vi "WFDC Messenger Template.vi"() -> (15 "Error Out":errorcluster)   [LabVIEW 2020]
uses:
  <vilib>/vision/Image Controls.llb/IMAQ Image.ctl
  WFDC Controls/WFDC Actions.ctl
  WFDC Controls/WFDC Notifier Element.ctl
  WFDC Controls/WFDC Status.ctl
  WFDC Controls/WFDC Cycle Pause.ctl
  WFDC Controls/WFDC External Sync.ctl
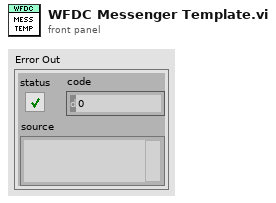
[diagram p1: front panel]
types:
  T1 = typedef "WFDC Notifier Element.ctl" = cluster{"WFDC Actions":T2, "Initial XYZ Positions":dbl[], "Ref Images":T3[], "Calibration (slope, inter)":dbl[], "Base Path":path, "Latest Scan Path":path, "Error":errorcluster, "XYZ Drift":dbl[]}
  T2 = typedef "WFDC Actions.ctl" = enum16{"Error Check", "Remote Start", "Move to Pos", "Pre Start Get Drift", "Pre Start Check Drift", "Pre Start Z Drift", "Pre Start XY Drift", "Pre Start ReFocus", "Setup New DC", "Setup Camera", "Get Ref Images", "Calc Calibration", "Switch Tabs", "Get Drift", "Z Drift", "XY Drift", "Start Cycle", "Stop DC", "Abort Remote", "Exit Loop", "Set Error", "Generate Calibration", "Quit"}
  T3 = typedef "IMAQ Image.ctl" = refnum<image>
  T4 = typedef "WFDC External Sync.ctl" = cluster{"Cycle Sync":T5, "Z Offset":dbl, "WFDC Status":T6}
  T5 = typedef "WFDC Cycle Pause.ctl" = enum16{"Pause Requested", "Paused", "Resume Requested", "Resumed"}
  T6 = typedef "WFDC Status.ctl" = enum16{"Idle", "Busy", "DC Active", "Error", "Canceled"}
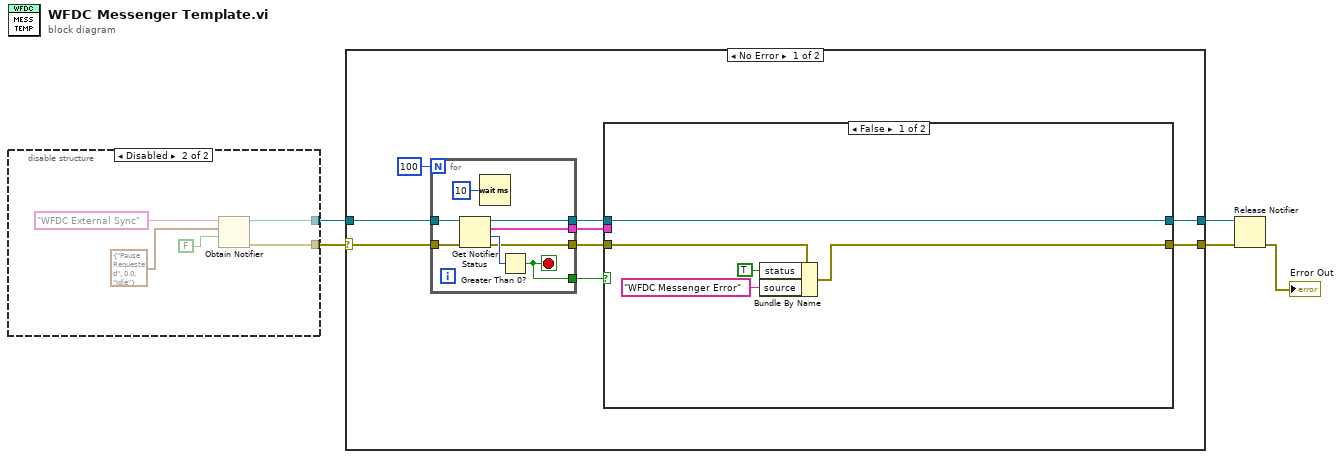
[diagram p0: block diagram]
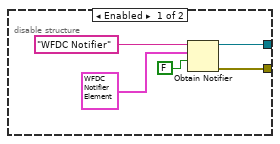
[diagram p2: hidden frame]
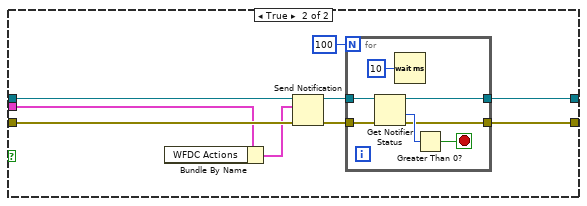
[diagram p3: hidden frame]
diagram:
  n1 = disable-structure shown="Disabled" {
    disable-tunnel: [w7 w12] -> w2
    disable-tunnel: [w6 w11] -> w1
    frame Enabled {
      n2 = Obtain Notifier(name (unnamed)="WFDC Notifier", notification data type=T1 {"WFDC Actions"=enum."Error Check", "Initial XYZ Positions"=[], "Ref Images"=[], "Calibration (slope, inter)"=[], "Base Path"=path "", "Latest Scan Path"=path "", "Error"={"status"=FALSE, "code"=0, "source"=""}, "XYZ Drift"=[]} ("WFDC Notifier Element"), create if not found? (T)=FALSE) -> (notifier out=w7:refnum<notifier>, error out=w6:errorcluster)  [unwired: 1 in, 1 out]
    }
    frame Disabled {
      n3 = Obtain Notifier(name (unnamed)="WFDC External Sync", notification data type=T4 {"Cycle Sync"=enum."Pause Requested", "Z Offset"=0.0, "WFDC Status"=enum."Idle"} ("WFDC External Sync"), create if not found? (T)=FALSE) -> (notifier out=w12:refnum<notifier>, error out=w11:errorcluster)  [unwired: 1 in, 1 out]
    }
  }
  n4 = case shown="No Error" w1 {
    selector: w1 -> [w22 w54]
    tunnel: w2 -> [w23 w55]
    tunnel: [w17 w55] -> w5
    tunnel: [w16 w54] -> w4
    frame No Error {
      n5 = for {
        N: 100 -> [_]
        tunnel: w23 -> [w52]
        tunnel: w22 -> [w51]
        tunnel: [w49] -> w20
        tunnel: [w48] -> w19
        tunnel: [w47] -> w21
        tunnel: [w46] -> w18
        stop <- w47 stop-if-true
        n6 = Get Notifier Status(notifier=w52, error in (no error)=w51) -> (notifier out=w49:refnum<notifier>, current notification=w46:T1, # waiting=w50:i32, error out=w48:errorcluster)  [unwired: 1 out]
        n7 = Wait (ms)(milliseconds to wait=u32 10) -> ()  [unwired: 1 out]
        n8 = Greater Than 0?(x=w50) -> (x > 0?=w47:bool)
      }
      n9 = case shown="False" w21 {
        tunnel: w20 -> [w29 w38]
        tunnel: w19 -> [w28 w37]
        tunnel: w18 -> [_ w31]
        tunnel: [w29 w33] -> w17
        tunnel: [w25 w32] -> w16
        frame False {
          n10 = Bundle By Name(cluster=w28, "status"=TRUE, "source"="WFDC Messenger Error") -> (w25:errorcluster)
        }
        frame True {
          n11 = Bundle By Name(cluster=w31) -> (w30:T1)  [unwired: 1 in]
          n12 = Send Notification(notification=w30, notifier=w38, error in (no error)=w37) -> (notifier out=w35:refnum<notifier>, error out=w34:errorcluster)
          n13 = for {
            N: 100 -> [_]
            tunnel: w35 -> [w44]
            tunnel: w34 -> [w43]
            tunnel: [w41] -> w33
            tunnel: [w40] -> w32
            stop <- w39 stop-if-true
            n14 = Get Notifier Status(notifier=w44, error in (no error)=w43) -> (notifier out=w41:refnum<notifier>, # waiting=w42:i32, error out=w40:errorcluster)  [unwired: 2 out]
            n15 = Wait (ms)(milliseconds to wait=u32 10) -> ()  [unwired: 1 out]
            n16 = Greater Than 0?(x=w42) -> (x > 0?=w39:bool)
          }
        }
      }
    }
    frame Error {
    }
  }
  n17 = Release Notifier(notifier=w5, error in (no error)=w4) -> (error out=→"Error Out":errorcluster)  [unwired: 1 in, 2 out]
